vi "Get Element.vi"(8 "error in (no error)":errorcluster caption="entrée d'erreur (pas d'erreur)", 10 "nom":string, 11 "Container en entrée":refnum<class "Container.lvclass">) -> (0 "error out":errorcluster caption="sortie d'erreur", 2 "données":refnum<class "Parent.lvclass">, 3 "Container en sortie":refnum<class "Container.lvclass">)   [LabVIEW 2015, in "Container.lvclass"]
uses:
  Container.lvclass
  Parent/Parent.lvclass
  Container.lvclass/Container.ctl
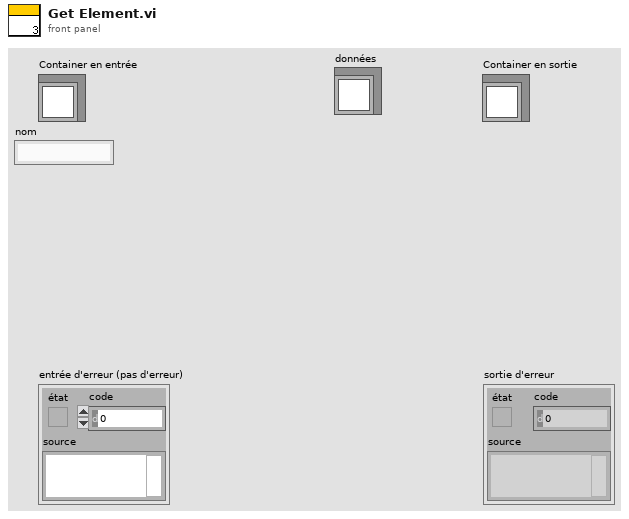
[diagram p1: front panel]
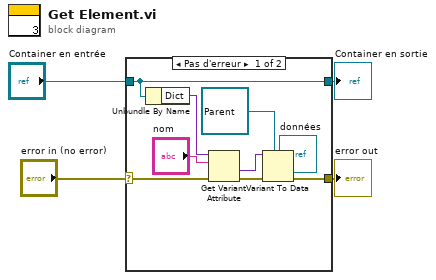
[diagram p0: block diagram]
diagram:
  n1 = case shown="Pas d'erreur" "error in (no error)" {
    selector: "error in (no error)" -> [w7 w15]
    tunnel: [w6 w15] -> w3
    tunnel: [w13 w14] -> w1
    tunnel: "Container en entrée" -> [w13 w14]
    frame No Error {
      n2 = Unbundle By Name(w13) -> ("Dict"=w12:variant)
      n3 = Get Variant Attribute(Variant=w12, name="nom", error in=w7) -> (value=w9:variant, error out=w8:errorcluster)  [unwired: 1 in, 2 out]
      n4 = Variant To Data(error in=w8, type=refnum<class "Parent.lvclass"> refnum ("Parent.lvclass"), Variant=w9) -> (data=→"données":refnum<class "Parent.lvclass">, error out=w6:errorcluster)
    }
    frame Error {
    }
  }
  "error out" <- w3
  "Container en sortie" <- w1
